vi "Settings Page.vi"() -> ()   [LabVIEW 2018, in "Protocols.lvlib" / "TCP.lvclass"]
uses:
  TCP.lvclass
panel:
  in  "Protocol Settings":enum32{"TCP/IP"}(tab)
  in  "Port":u16
  in  "IP Address":string="localhost"
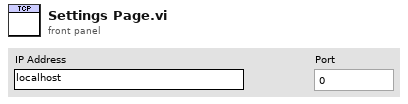
[diagram p1: front panel]
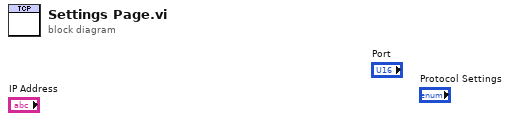
[diagram p0: block diagram]
diagram:
